vi "Initialise.vi"(2 "error in (no error)":errorcluster, 3 "Bounds":dbl[](array[numeric])) -> (0 "error out":errorcluster, 1 "Rectangle.lvclass":refnum<class "Rectangle.lvclass">)   [LabVIEW 2015, in "Rectangle.lvclass"]
uses:
  Rectangle.lvclass
  Rectangle.lvclass/Rectangle.ctl
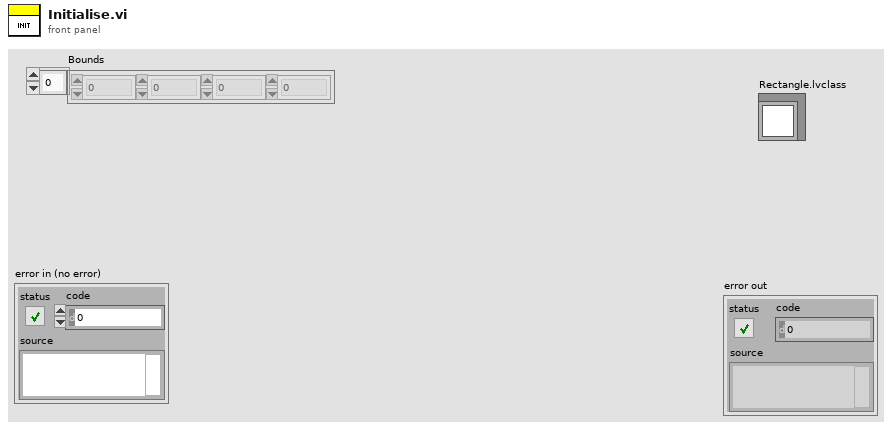
[diagram p1: front panel]
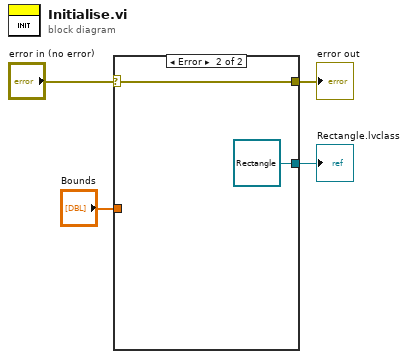
[diagram p0: block diagram]
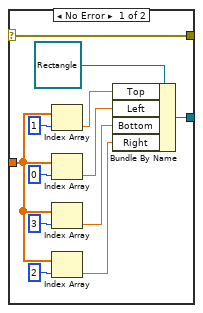
[diagram p2: hidden frame]
diagram:
  n1 = case shown="Error" "error in (no error)" {
    selector: "error in (no error)" -> [w16 w18]
    tunnel: [w16 w18] -> w3
    tunnel: "Bounds" -> [w11 _]
    tunnel: [w5 refnum<class "Rectangle.lvclass"> refnum ("Rectangle.lvclass")] -> w1
    frame No Error {
      n2 = Index Array(array=w11, index=1) -> (element=w8:dbl)
      n3 = Index Array(array=w11, index=0) -> (element=w9:dbl)
      n4 = Index Array(array=w11, index=3) -> (element=w6:dbl)
      n5 = Index Array(array=w11, index=2) -> (element=w7:dbl)
      n6 = Bundle By Name(cluster=refnum<class "Rectangle.lvclass"> refnum ("Rectangle.lvclass"), "Top"=w8, "Left"=w9, "Bottom"=w6, "Right"=w7) -> (w5:refnum<class "Rectangle.lvclass">)
    }
    frame Error {
    }
  }
  "error out" <- w3
  "Rectangle.lvclass" <- w1
